vi "String to Array.vi"(11 "Data":string="currentLimit[01]=0\r\ncurrentLimit[02]=0\r\ncurrentLimit[03]=0\r\ncurrentLimit[04]=0\r\ncurrentLimit[05]=0\r\ncurrentLimit[06]=0\r\ncurrentLimit[07]=0\r\ncurrentLimit[08]=0\r\ncurrentLimit[09]=0\r\ncurrentLimit[10]=0\r\ncurrentLimit[11]=0\r\ncurrentLimit[12]=0\r\ncurrentLimit[13]=0\r\ncurrentLimit[14]=0\r\ncurrentLimit[15]=0\r\ncurrentLimit[16]=0\r\ncurrentLimit[17]=0\r\ncurrentLimit[18]=0\r\ncurrentLimit[19]=0\r\ncurrentLimit[20]=0\r\ncurrentLimit[21]=0\r\ncurrentLimit[22]=0\r\ncurrentLimit[23]=0\r\ncurrentLimit[24]=0\r\ncurrentLimit[25]=0\r\ncurrentLimit[26]=0\r\nchargeLimit[01]=0\r\nchargeLimit[02]=0\r\nchargeLimit[03]=0\r\nchargeLimit[04]=0\r\nchargeLimit[05]=0\r\nchargeLimit[06]=0\r\nchargeLimit[07]=0\r\nchargeLimit[08]=0\r\nchargeLimit[09]=0\r\nchargeLimit[10]=0\r\nchargeLimit[11]=0\r\nchargeLimit[12]=0\r\nchargeLimit[13]=0\r\nchargeLimit[14]=0\r\nchargeLimit[15]=0\r\nchargeLimit[16]=0\r\nchargeLimit[17]=0\r\nchargeLimit[18]=0\r\nchargeLimit[19]=0\r\nchargeLimit[20]=0\r\nchargeLimit[21]=0\r\nchargeLimit[22]=0\r\nchargeLimit[23]=0\r\nchargeLimit[24]=0\r\nchargeLimit[25]=0\r\nchargeLimit[26]=0") -> (2 "chargeLimit":i32[](array[numeric]), 3 "currentLimit":i32[](array[numeric]))   [LabVIEW 2010]
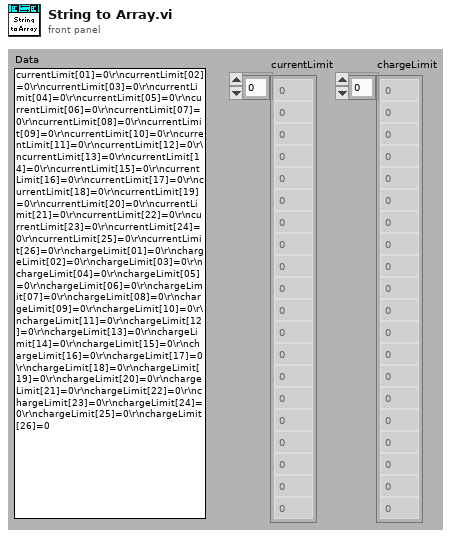
[diagram p1: front panel]
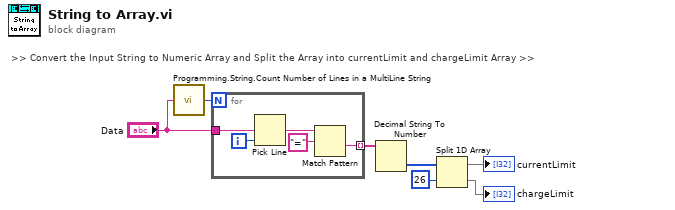
[diagram p0: block diagram]
diagram:
  # ">> Convert the Input String to Numeric Array and Split the Array into currentLimit and chargeLimit Array >>"
  n1 = call "Programming.String.Count Number of Lines in a MultiLine String.vi"("MultiLine String Input"="Data") -> ("Number of Lines"=w5:i32)  [unwired: 4 in]
  n2 = for {
    N: w5 -> [_]
    tunnel: "Data" -> [w8]
    tunnel: [w9] -> w4 mode=indexing
    i -> [w11]
    n3 = Pick Line(multi-line string=w8, line index=w11) -> (output string=w10:string)  [unwired: 1 in]
    n4 = Match Pattern(string=w10, regular expression="=") -> (after substring=w9:string)  [unwired: 1 in, 3 out]
  }
  n5 = Decimal String To Number(string=w4) -> (number=w3:i32[])  [unwired: 2 in, 1 out]
  n6 = Split 1D Array(array=w3, index=26) -> (first subarray=→"currentLimit":i32[], second subarray=→"chargeLimit":i32[])
